vi "detector-andor-xenics-switch.vi"(1 "Detector":u16(ring) caption="Camera" items=["Newton", "iDus", "Clara", "Xeva"]) -> (0 "Manufacturer":enum16{"Andor", "Xenics", "unknown"}(ring))   [LabVIEW 2015]
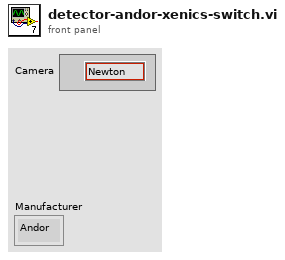
[diagram p1: front panel]
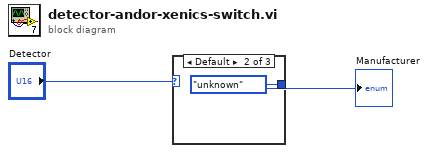
[diagram p0: block diagram]
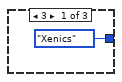
[diagram p2: hidden frame]
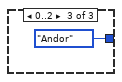
[diagram p3: hidden frame]
diagram:
  n1 = case shown="Default" "Detector" {
    tunnel: [enum16{"Andor", "Xenics"}."Xenics" ("Manufacturer") enum16{"Andor", "Xenics", "unknown"}."unknown" ("Manufacturer") enum16{"Andor", "Xenics"}."Andor" ("Manufacturer")] -> w2
    frame 3 {
    }
    frame Default {
    }
    frame 0..2 {
    }
  }
  "Manufacturer" <- w2
